vi "test_Set-Get Instrument Addon Name.vi"(8 "error in (no error)":errorcluster, 11 "TestCase in":refnum<class "Instrument Addon Scripting API Custom Device Unit Tests.lvclass">) -> (0 "error out":errorcluster, 3 "TestCase out":refnum<class "Instrument Addon Scripting API Custom Device Unit Tests.lvclass">)   [LabVIEW 2018, in "Instrument Addon Scripting API Custom Device Unit Tests.lvclass"]
uses:
  Instrument Addon Scripting API Custom Device Unit Tests.lvclass
  <vilib>/addons/_JKI Toolkits/VI Tester/TestCase.llb/TestCase.lvclass
  Instrument Addon Scripting API Test Assets/Instrument Addon Scripting API Test Assets.lvclass
  APIs/Scripting API/Instrument Addon Scripting API.lvlib
  C:/Program Files (x86)/National Instruments/LabVIEW 2018/vi.lib/addons/_JKI Toolkits/VI Tester/TestCase.llb/TestCase.lvclass
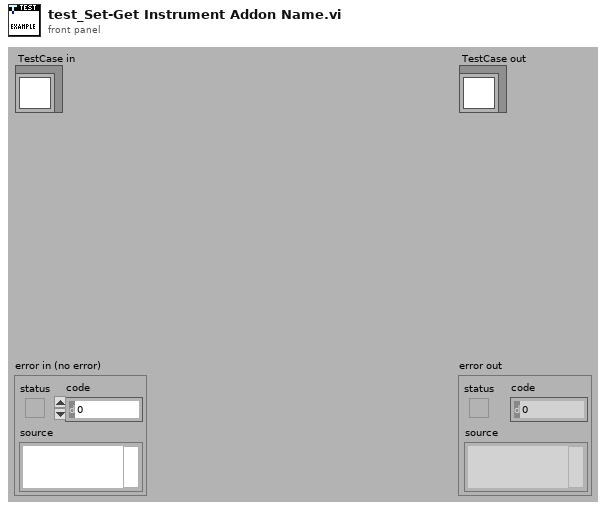
[diagram p1: front panel]
types:
  T1 = typedef "Custom Device API.lvlib/Custom Device Item Ref.ctl" = u64
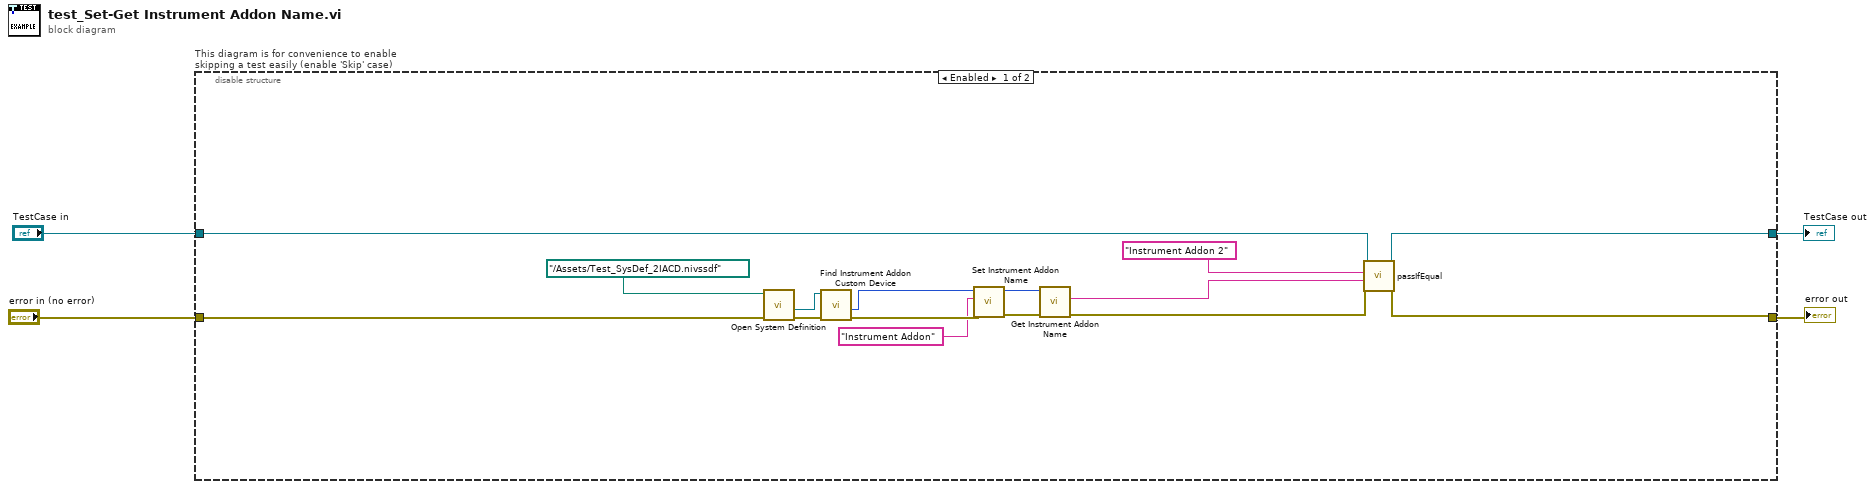
[diagram p0: block diagram]
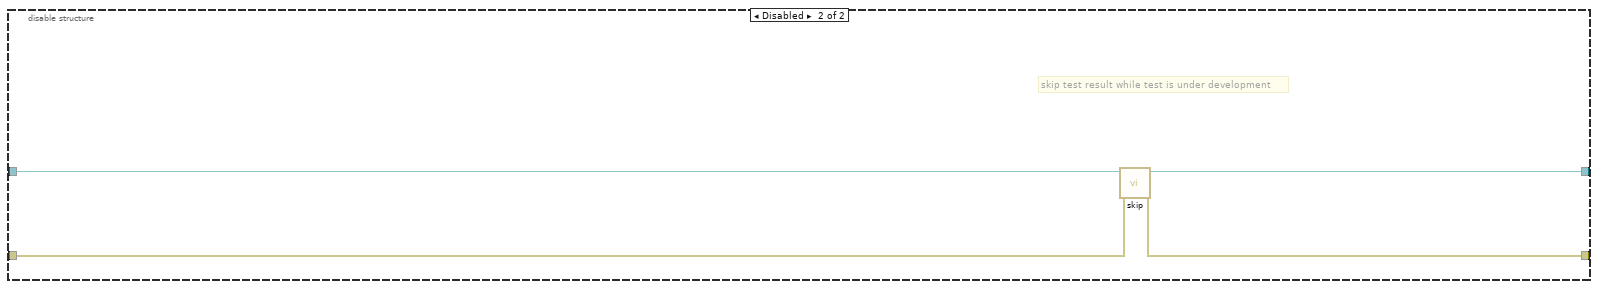
[diagram p2: hidden frame]
diagram:
  n1 = disable-structure "This diagram is for convenience to enable skipping a test easily (enable 'Skip' case)" shown="Enabled" {
    disable-tunnel: "TestCase in" -> [w19 w23]
    disable-tunnel: [w18 w21] -> w1
    disable-tunnel: [w17 w22] -> w3
    disable-tunnel: "error in (no error)" -> [w16 w20]
    frame Enabled {
      n2 = call "Open System Definition.vi"("error in (no error)"=w16, "System Definition File"=path "../Assets/Test_SysDef_2IACD.nivssdf") -> ("error out"=w15:errorcluster, "Target Refnum"=w14:refnum<k24>)  [unwired: 6 in, 2 out]
      n3 = call "Find Instrument Addon Custom Device.vi"("error in"=w15, "target in"=w14) -> ("error out"=w13:errorcluster, "NodeID"=w12:u64)  [unwired: 7 in, 1 out]
      n4 = call "Set Instrument Addon Name.vi"("Error In"=w13, "Name"="Instrument Addon", "Instrument Addon Refnum In"=w12) -> ("Error Out"=w9:errorcluster, "Instrument Addon Refnum Out"=w8:T1)  [unwired: 7 in]
      n5 = call "Get Instrument Addon Name.vi"("Error In"=w9, "Instrument Addon Refnum In"=w8) -> ("Error Out"=w6:errorcluster, "Name"=w7:string)  [unwired: 7 in, 1 out]
      n6 = call-dynamic "passIfEqual.vi"("error in (no error)"=w6, "y"=w7, "x"="Instrument Addon 2", "TestCase in"=w19) -> ("error out"=w17:errorcluster, "TestCase out"=w18:refnum<class "Instrument Addon Scripting API Custom Device Unit Tests.lvclass">)  [unwired: 6 in]
    }
    frame Disabled {
      # "skip test result while test is under development"
      n7 = call <vilib>:"skip.vi"("error in (no error)"=w20, "TestCase in"=w23) -> ("error out"=w22:errorcluster, "TestCase out"=w21:refnum<class "Instrument Addon Scripting API Custom Device Unit Tests.lvclass">)  [unwired: 8 in]
    }
  }
  "error out" <- w3
  "TestCase out" <- w1
